vi "3-element-Linearization.vi"(6 "B":i32, 7 "C3":i32, 9 "Voltage in":dbl, 10 "C1":i32, 11 "C2":i32) -> (3 "Scaled value":dbl)   [LabVIEW 2020]
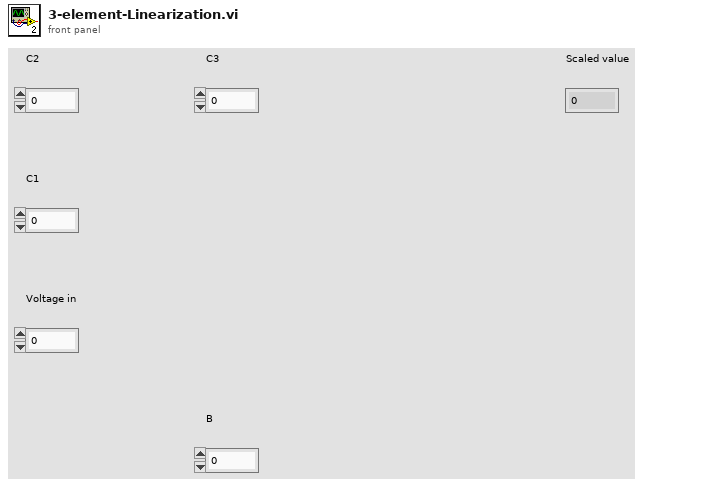
[diagram p1: front panel]
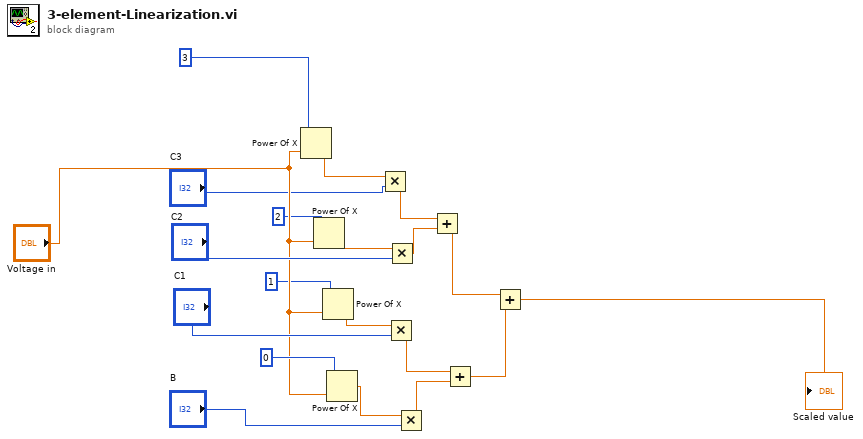
[diagram p0: block diagram]
diagram:
  n1 = Power Of X(1:"Voltage in", 2:3) -> (0:w4:dbl)
  n2 = Power Of X(1:"Voltage in", 2:2) -> (0:w9:dbl)
  n3 = Power Of X(1:"Voltage in", 2:1) -> (0:w11:dbl)
  n4 = Power Of X(1:"Voltage in", 2:0) -> (0:w13:dbl)
  n5 = Multiply(x=w4, y="C3") -> (x*y=w16:dbl)
  n6 = Multiply(x=w11, y="C1") -> (x*y=w18:dbl)
  n7 = Multiply(x=w9, y="C2") -> (x*y=w15:dbl)
  n8 = Multiply(x=w13, y="B") -> (x*y=w17:dbl)
  n9 = Add(x=w16, y=w15) -> (x+y=w20:dbl)
  n10 = Add(x=w18, y=w17) -> (x+y=w19:dbl)
  n11 = Add(x=w20, y=w19) -> (x+y=→"Scaled value":dbl)
